vi "Global.vi"() -> ()   [LabVIEW 2016]
panel:
  out "delay":i32
  in  "w2":i32 min=0 max=3000 step=1
  in  "h2":i32 min=0 max=3000 step=1
  in  "w1":i32 min=0 max=3000 step=1
  in  "h1":i32 min=0 max=3000 step=1
  out "actual":dbl
  out "frames_rec":i32
  in  "stop":bool
  out "moving":bool
  out "cam_status":bool
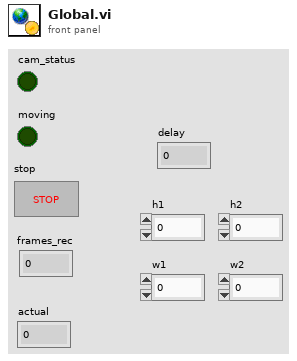
[diagram p1: front panel]
diagram:
